vi "Set Graphs to Default.vi"(11 "Array":refnum<vi>[](array[refnum])) -> ()   [LabVIEW 2019, in "CML UI.lvlib"]
uses:
  CML UI.lvlib
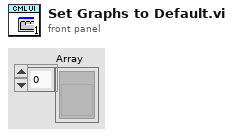
[diagram p1: front panel]
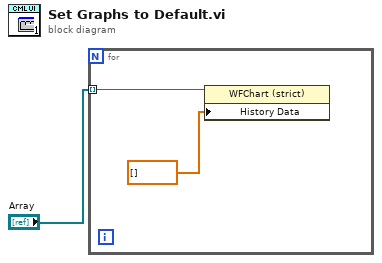
[diagram p0: block diagram]
diagram:
  n1 = for {
    tunnel: "Array" -> [w3] mode=indexing
    n2 = property class="WFChart (strict)"(reference=w3, "History Data"=dbl[] []) -> ()  [unwired: 1 in, 2 out]
  }
